vi "Selection In Tree.vi"(10 "Tree":string(tree)) -> (2 "Selected item":string)   [LabVIEW 2017]
panel:
  in  "Done":bool
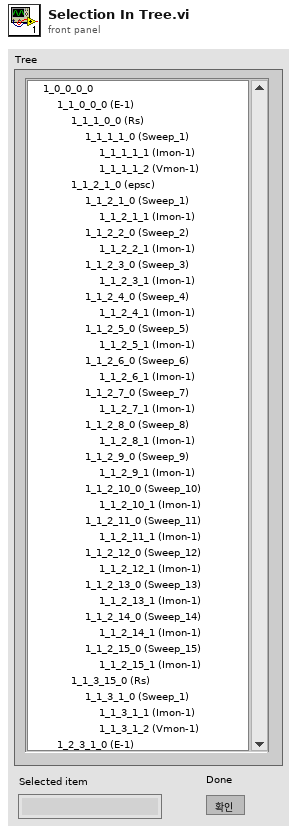
[diagram p1: front panel]
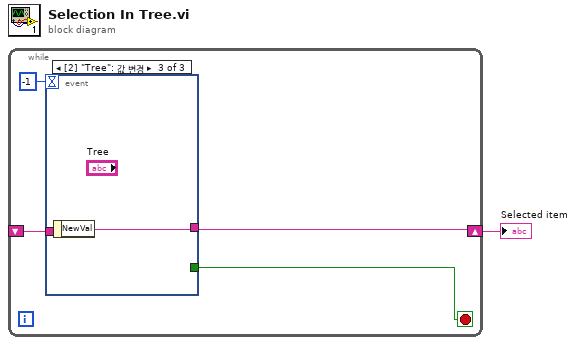
[diagram p0: block diagram]
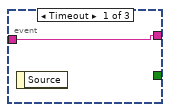
[diagram p2: hidden frame]
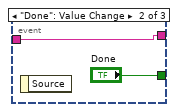
[diagram p3: hidden frame]
diagram:
  n1 = while {
    shift-right: [w4] -> w1
    shift-left: _ -> [w3]
    stop <- w5 stop-if-true
    n2 = event shown="[2] \"Tree\": 값 변경" {
      selector: _ -> [_ _ _]
      dyn-events: _ -> [_ _ _]
      timeout: -1 -> [_ _ _]
      tunnel: [_ "Done" _] -> w5
      tunnel: [w6 w7 w9] -> w4
      tunnel: w3 -> [w6 w7 _]
      event Timeout {
        n3 = event-data() -> ()  [unwired: 1 in, 1 out]
      }
      event "Done": Value Change {
        n4 = event-data() -> ()  [unwired: 1 in, 1 out]
      }
      event "Tree": Value Change {
        n5 = event-data() -> ("NewVal"=w9:string)  [unwired: 1 in]
      }
    }
  }
  "Selected item" <- w1
